vi "GV_ZoomWindowPerform.vi"(8 "error in (no error)":errorcluster, 9 "Coords":T1, 11 "Gviewer in":refnum<class "Gviewer.lvclass">) -> (0 "error out":errorcluster, 3 "Gviewer out":refnum<class "Gviewer.lvclass">)   [LabVIEW 2020, in "Sgraph_lib_V1.lvlib" / "Gviewer.lvclass"]
doc: "Andre Koelewijn, 5 may 2021\n\nPerform the window zoom action when the mouse button is released"
uses:
  Gviewer.lvclass
  <vilib>/Utility/miscctls.llb/LVPoint32TypeDef.ctl
  Gviewer.lvclass/Gviewer.ctl
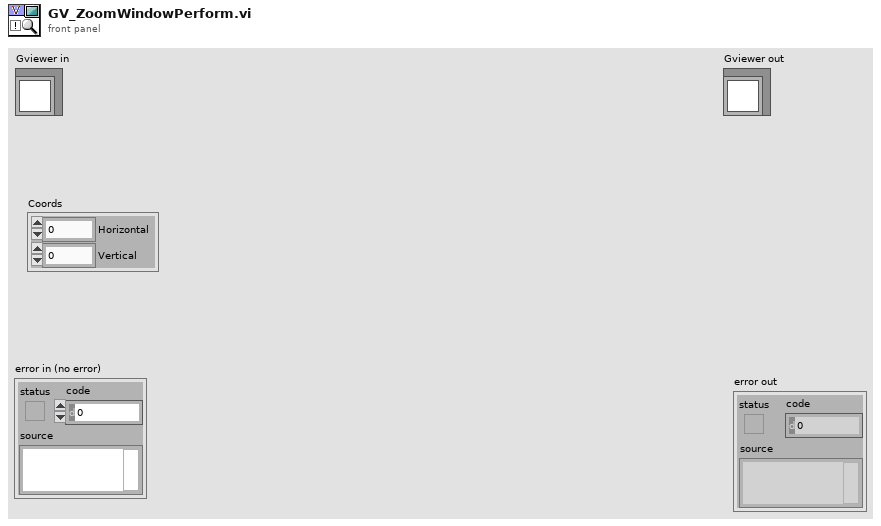
[diagram p1: front panel]
types:
  T1 = typedef "LVPoint32TypeDef.ctl" = cluster{"Horizontal":i32, "Vertical":i32}
  T2 = cluster{"left":i16, "top":i16, "right":i16, "bottom":i16}
  T3 = typedef "Sgraph_lib_V1.lvlib/Gviewer.lvclass/Typedef_SelProperties.ctl" = cluster{"Color":u32, "LineType":T4, "max":dbl, "min":dbl, "unit":string}
  T4 = typedef "Sgraph_lib_V1.lvlib/Gviewer.lvclass/Typedef_LineType.ctl" = enum16{"num_bare", "num_MinMax_Area", "num_MinMax_Lines", "num_MinMax_Forfor", "num_Max_Area", "num_Max_Line", "num_Max_Forfor", "num_Min_Area", "num_Min_Line", "num_Min_Fosfor", "Boolean_Line_01", "Boolean_Area_01", "Boolean_Fosfor_01", "Boolean_Line_TF", "Boolean_Area_TF", "Boolean_Fosfor_TF", "Boolean_OnOff_Line", "Boolean_OnOff_Area", "Boolean_OnOff_Fosfor", "Boolean_spare", "StringEvent_Line", "StringEvent_TimeLine"}
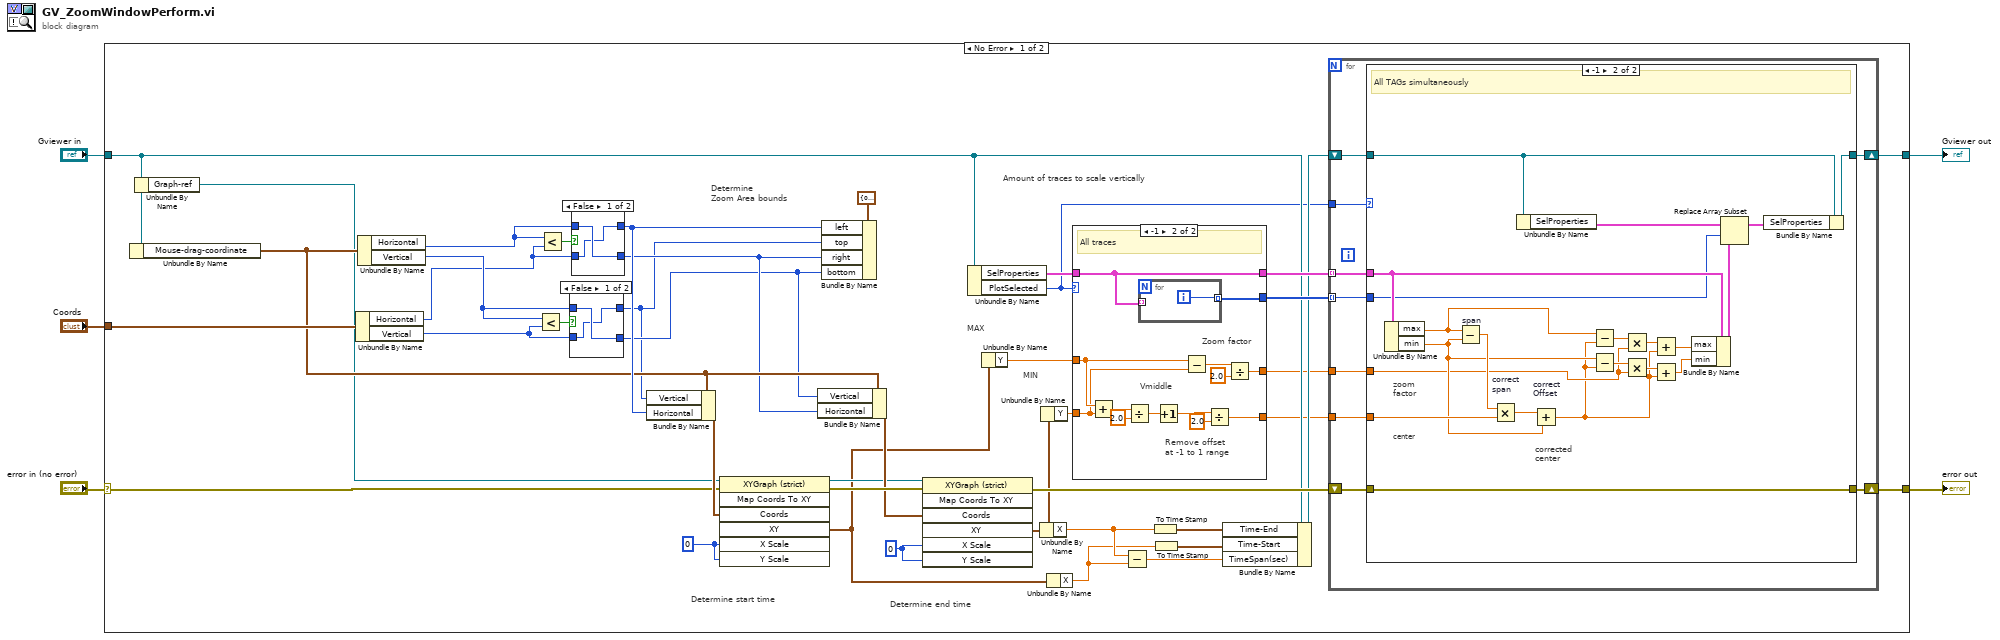
[diagram p0: block diagram]
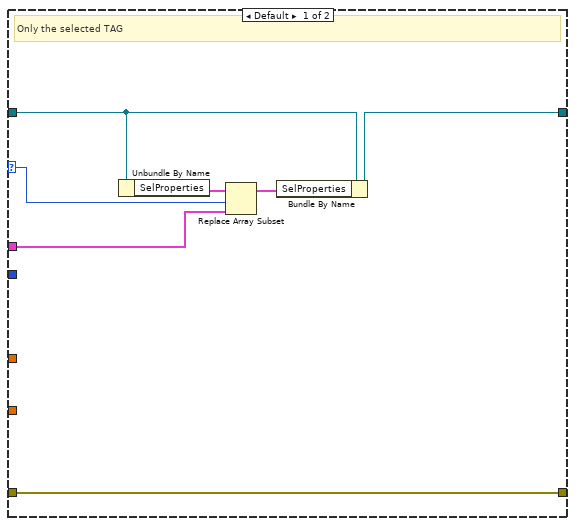
[diagram p2: hidden frame]
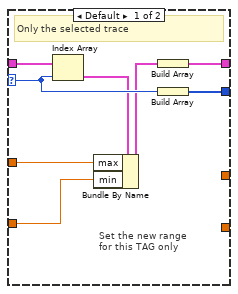
[diagram p3: hidden frame]
diagram:
  n1 = case shown="No Error" "error in (no error)" {
    selector: "error in (no error)" -> [w6 w115]
    tunnel: [w27 w115] -> w4
    tunnel: [w26 w114] -> w2
    tunnel: "Gviewer in" -> [w21 w114]
    tunnel: "Coords" -> [w31 _]
    frame No Error {
      w39 = 0 ("X Scale")
      w38 = 0 ("X Scale")
      # "MAX"
      # "MIN"
      # "Amount of traces to scale vertically"
      # "Determine\nZoom Area bounds"
      # "Determine start time"
      # "Determine end time"
      n2 = Unbundle By Name(w21) -> ("Mouse-drag-coordinate"=w25:T1)
      n3 = Unbundle By Name(w21) -> ("Graph-ref"=w7:refnum<vi>)
      n4 = Unbundle By Name(w31) -> ("Horizontal"=w12:i32, "Vertical"=w11:i32)
      n5 = Unbundle By Name(w25) -> ("Horizontal"=w14:i32, "Vertical"=w13:i32)
      n6 = Less?(x=w13, y=w11) -> (x < y?=w41:bool)
      n7 = Less?(x=w14, y=w12) -> (x < y?=w40:bool)
      n8 = case shown="False" w41 {
        tunnel: w13 -> [w107 w109]
        tunnel: [w106 w109] -> w15
        tunnel: [w107 w108] -> w16
        tunnel: w11 -> [w106 w108]
        frame False {
        }
        frame True {
        }
      }
      n9 = case shown="False" w40 {
        tunnel: w14 -> [w111 w113]
        tunnel: [w110 w113] -> w46
        tunnel: [w111 w112] -> w23
        tunnel: w12 -> [w110 w112]
        frame False {
        }
        frame True {
        }
      }
      n10 = Bundle By Name(cluster=w25, "Vertical"=w15, "Horizontal"=w46) -> (w42:T1)
      n11 = invoke class="XYGraph (strict)" method="Map Coords To XY"(reference=w7, error in=w6, "Coords"=w42, "X Scale"=w38, "Y Scale"=w38) -> (reference out=w43:refnum<vi>, error out=w45:errorcluster, "XY"=w18:cluster{"X":dbl, "Y":dbl})  [unwired: 2 in, 4 out]
      n12 = Bundle By Name(cluster=w25, "Vertical"=w16, "Horizontal"=w23) -> (w44:T1)
      n13 = Bundle By Name(cluster=T2 {"left"=0, "top"=0, "right"=0, "bottom"=0} ("rect"), "left"=w46, "top"=w15, "right"=w23, "bottom"=w16) -> ()  [unwired: 1 out]
      n14 = invoke class="XYGraph (strict)" method="Map Coords To XY"(reference=w43, error in=w45, "Coords"=w44, "X Scale"=w39, "Y Scale"=w39) -> (error out=w28:errorcluster, "XY"=w20:cluster{"X":dbl, "Y":dbl})  [unwired: 2 in, 5 out]
      n15 = Unbundle By Name(w21) -> ("SelProperties"=w30:T3[], "PlotSelected"=w8:i32)
      n16 = Unbundle By Name(w18) -> ("Y"=w17:dbl)
      n17 = Unbundle By Name(w20) -> ("X"=w35:dbl)
      n18 = Unbundle By Name(w20) -> ("Y"=w19:dbl)
      n19 = Unbundle By Name(w18) -> ("X"=w34:dbl)
      n20 = case shown="-1" w8 {
        selector: w8 -> [w89 _]
        tunnel: w30 -> [w90 w103]
        tunnel: [w91 w103] -> w24
        tunnel: [w88 w104] -> w29
        tunnel: w19 -> [w84 w95]
        tunnel: w17 -> [w85 w96]
        tunnel: [_ w97] -> w10
        tunnel: [_ w92] -> w9
        frame Default {
          # "Set the new range\nfor this TAG only"
          # "Only the selected trace"
          n21 = Index Array(array=w90, index=w89) -> (element=w87:T3)
          n22 = Bundle By Name(cluster=w87, "max"=w85, "min"=w84) -> (w86:T3)
          n23 = Build Array(w86) -> (w91:T3[])
          n24 = Build Array(w89) -> (w88:i32[])
        }
        frame -1 {
          # "Zoom factor"
          # "Remove offset\nat -1 to 1 range"
          # "Vmiddle"
          # "All traces"
          n25 = Add(x=w96, y=w95) -> (x+y=w102:dbl)
          n26 = Divide(x=w102, y=2.0) -> (x/y=w100:dbl)
          n27 = for {
            tunnel: [w105] -> w104 mode=indexing
            tunnel: w103 -> [_] mode=indexing
            i -> [w105]
          }
          n28 = Increment ("remove offset\nat -1 to 1 range")(x=w100) -> (x+1=w98:dbl)
          n29 = Subtract(x=w96, y=w95) -> (x-y=w93:dbl)
          n30 = Divide(x=w98, y=2.0) -> (x/y=w97:dbl)
          n31 = Divide(x=w93, y=2.0) -> (x/y=w92:dbl)
        }
      }
      n32 = Subtract(x=w35, y=w34) -> (x-y=w36:dbl)
      n33 = To Time Stamp(1:w35) -> (0:w32:timestamp)
      n34 = To Time Stamp(1:w34) -> (0:w33:timestamp)
      n35 = Bundle By Name(cluster=w21, "Time-End"=w32, "Time-Start"=w33, "TimeSpan(sec)"=w36) -> (w22:refnum<class "Gviewer.lvclass">)
      n36 = for {
        tunnel: w24 -> [w53] mode=indexing
        tunnel: w29 -> [w48] mode=indexing
        shift-right: [w54] -> w26
        shift-left: w22 -> [w55]
        shift-right: [w51] -> w27
        shift-left: w28 -> [w52]
        tunnel: w10 -> [w50]
        tunnel: w9 -> [w49]
        tunnel: w8 -> [w47]
        n37 = case shown="-1" w47 {
          selector: w47 -> [w60 _]
          tunnel: w55 -> [w62 w81]
          tunnel: [w61 w80] -> w54
          tunnel: w53 -> [w59 w64]
          tunnel: w52 -> [w58 w79]
          tunnel: [w58 w79] -> w51
          tunnel: w50 -> [_ w78]
          tunnel: w49 -> [_ w71]
          tunnel: w48 -> [_ w63]
          frame Default {
            # "Only the selected TAG"
            n38 = Unbundle By Name(w62) -> ("SelProperties"=w56:T3[])
            n39 = Replace Array Subset(array=w56, new element=w59, index=w60) -> (w57:T3[])
            n40 = Bundle By Name(cluster=w62, "SelProperties"=w57) -> (w61:refnum<class "Gviewer.lvclass">)
          }
          frame -1 {
            # "corrected\ncenter"
            # "zoom\nfactor"
            # "center"
            # "All TAGs simultaneously"
            n41 = Unbundle By Name(w64) -> ("max"=w75:dbl, "min"=w74:dbl)
            n42 = Subtract "span"(x=w75, y=w74) -> (x-y=w77:dbl)
            n43 = Multiply "correct\nspan"(x=w77, y=w78) -> (x*y=w76:dbl)
            n44 = Unbundle By Name(w81) -> ("SelProperties"=w82:T3[])
            n45 = Add "correct\nOffset"(x=w76, y=w74) -> (x+y=w68:dbl)
            n46 = Subtract(x=w75, y=w68) -> (x-y=w72:dbl)
            n47 = Subtract(x=w74, y=w68) -> (x-y=w73:dbl)
            n48 = Multiply(x=w72, y=w71) -> (x*y=w70:dbl)
            n49 = Multiply(x=w73, y=w71) -> (x*y=w69:dbl)
            n50 = Add(x=w70, y=w68) -> (x+y=w67:dbl)
            n51 = Add(x=w69, y=w68) -> (x+y=w66:dbl)
            n52 = Bundle By Name(cluster=w64, "max"=w67, "min"=w66) -> (w65:T3)
            n53 = Replace Array Subset(array=w82, new element=w65, index=w63) -> (w83:T3[])
            n54 = Bundle By Name(cluster=w81, "SelProperties"=w83) -> (w80:refnum<class "Gviewer.lvclass">)
          }
        }
      }
    }
    frame Error {
    }
  }
  "error out" <- w4
  "Gviewer out" <- w2
